vi "setWidget.vi"(8 "Error In":errorcluster, 10 "widget":refnum<class "QWidget.lvclass">, 11 "QScrollArea In":refnum<class "QScrollArea.lvclass">) -> (0 "Error Out":errorcluster, 3 "QScrollArea Out":refnum<class "QScrollArea.lvclass">)   [LabVIEW 2014, in "QScrollArea.lvclass"]
doc: "LabVIEW-specific documentation is not yet available. See <b>http://doc.qt.io/qt-5/QScrollArea.html#setWidget</b>"
uses:
  QScrollArea.lvclass
  QWidget/QWidget.lvclass
  LQ Core/LQIdentity/LQIdentity.lvclass/LQIdentity.ctl
  LQ Core/LQ Core.lvlib
  LQ Core/LQIdentity/LQIdentity.lvclass
panel:
  # "Copyright (c) 2016 Sze Howe Koh\n\nThis Source Code Form is subject to the terms of the Mozilla Public\nLicense, v. 2.0. If a copy of the MPL was not distributed with this\nfile, You can obtain one at http://mozilla.org/MPL/2.0/."
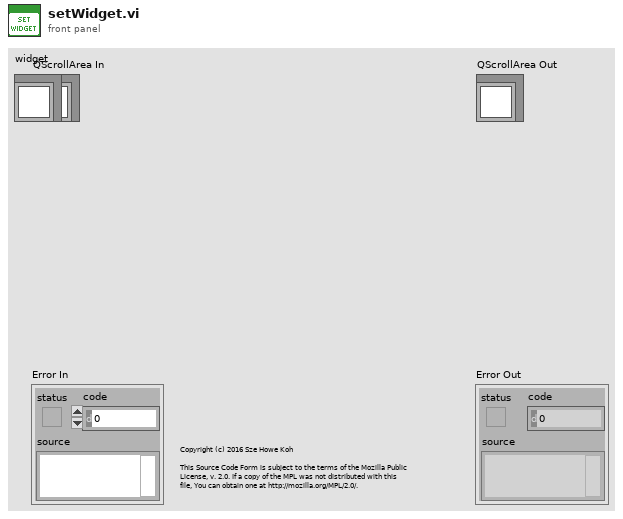
[diagram p1: front panel]
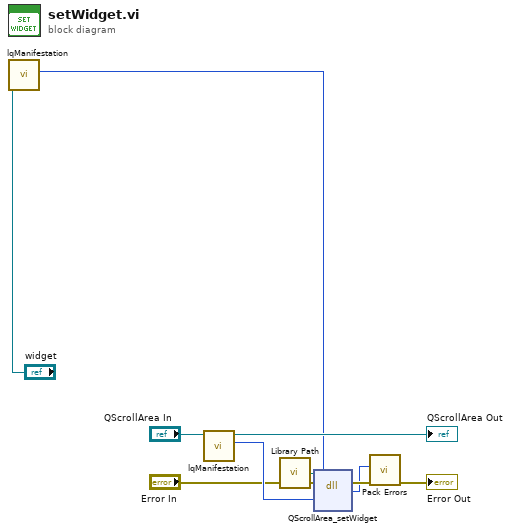
[diagram p0: block diagram]
diagram:
  n1 = call "lqManifestation.vi"("LQIdentity in"="widget") -> ("Manifestation"=w1:u64)  [unwired: 9 in, 1 out]
  n2 = call "lqManifestation.vi"("LQIdentity in"="QScrollArea In") -> ("Manifestation"=w7:u64, "LQIdentity out"=→"QScrollArea Out":refnum<class "QScrollArea.lvclass">)  [unwired: 9 in]
  n3 = call "Library Path.vi"() -> ("Library Path"=w8:path)
  n4 = dll-call lib="?" fn="QScrollArea_setWidget"(path in=w8, error in="Error In", "_instance"=w7, "widget"=w1) -> (error out=w5:errorcluster, w3:i32)  [unwired: 3 in, 1 out]
  n5 = call "Pack Errors.vi"("Error In"=w5, "Error Code"=w3) -> ("Error Out"=→"Error Out":errorcluster)  [unwired: 9 in]
